vi "VISJS Viewer.vi"(4 "Extra Scripts":string, 5 "FileDependency In":map{path, T1}(c390), 6 "Options":string, 7 "OpenWebBrowser(False)":bool, 8 "error in":errorcluster, 9 "Embedd VISJS Librarya in HTMl File(False)":bool, 10 "HTMLFilePath":path, 11 "LibraryDependency":map{path, T3}(c390)) -> (0 "error out":errorcluster, 3 "HTMLFileContent":string)   [LabVIEW 2020, in "VISJS Viewer.lvlib"] (continued)
,g)||A.deactivate()},document.body.addEventListener(\"click\",this._onClick),this._cleanupQueue.push((function(){document.body.removeEventListener(\"click\",A._onClick)}))),this._escListener=function(g){(\"key\"in g?\"Escape\"===g.key:27===g.keyCode)&&A.deactivate()}}He(jf.prototype),jf.current=null,jf.prototype.destroy=function(){var g,t;this.deactivate();var A,e=Rf(cl(g=Zl(t=this._cleanupQueue).call(t,0)).call(g));try{for(e.s();!(A=e.n()).done;){(0,A.value)()}}catch(g){e.e(g)}finally{e.f()}},jf.prototype.activate=function(){jf.current&&jf.current.deactivate(),jf.current=this,this.active=!0,this._dom.overlay.style.display=\"none\",this._dom.container.classList.add(\"vis-active\"),this.emit(\"change\"),this.emit(\"activate\"),document.body.addEventListener(\"keydown\",this._escListener)},jf.prototype.deactivate=function(){this.active=!1,this._dom.overlay.style.display=\"block\",this._dom.container.classList.remove(\"vis-active\"),document.body.removeEventListener(\"keydown\",this._escListener),this.emit(\"change\"),this.emit(\"deactivate\")},jf.prototype._onTapOverlay=function(g){this.activate(),g.srcEvent.stopPropagation()};var Lf=/^#?([a-f\\d]{2})([a-f\\d]{2})([a-f\\d]{2})$/i,Vf=/^#?([a-f\\d])([a-f\\d])([a-f\\d])$/i,Yf=/^rgb\\( *(1?\\d{1,2}|2[0-4]\\d|25[0-5]) *, *(1?\\d{1,2}|2[0-4]\\d|25[0-5]) *, *(1?\\d{1,2}|2[0-4]\\d|25[0-5]) *\\)$/i,Wf=/^rgba\\( *(1?\\d{1,2}|2[0-4]\\d|25[0-5]) *, *(1?\\d{1,2}|2[0-4]\\d|25[0-5]) *, *(1?\\d{1,2}|2[0-4]\\d|25[0-5]) *, *([01]|0?\\.\\d+) *\\)$/i;function Qf(g){if(g)for(;!0===g.hasChildNodes();){var t=g.firstChild;t&&(Qf(t),g.removeChild(t))}}function Uf(g){return g instanceof String||\"string\"==typeof g}function _f(g){return\"object\"===yd(g)&&null!==g}function Kf(g,t,A,e){var C=!1;!0===e&&(C=null===t[A]&&void 0!==g[A]),C?delete g[A]:g[A]=t[A]}function Hf(g,t){var A=arguments.length>2&&void 0!==arguments[2]&&arguments[2];for(var e in g)if(void 0!==t[e])if(null===t[e]||\"object\"!==yd(t[e]))Kf(g,t,e,A);else{var C=g[e],I=t[e];_f(C)&&_f(I)&&Hf(C,I,A)}}function Xf(g,t,A){var e=arguments.length>3&&void 0!==arguments[3]&&arguments[3];if(Rh(A))throw new TypeError(\"Arrays are not supported by deepExtend\");for(var C=0;C<g.length;C++){var I=g[C];if(Object.prototype.hasOwnProperty.call(A,I))if(A[I]&&A[I].constructor===Object)void 0===t[I]&&(t[I]={}),t[I].constructor===Object?qf(t[I],A[I],!1,e):Kf(t,A,I,e);else{if(Rh(A[I]))throw new TypeError(\"Arrays are not supported by deepExtend\");Kf(t,A,I,e)}}return t}function Jf(g,t,A){var e=arguments.length>3&&void 0!==arguments[3]&&arguments[3];if(Rh(A))throw new TypeError(\"Arrays are not supported by deepExtend\");for(var C in A)if(Object.prototype.hasOwnProperty.call(A,C)&&!Ic(g).call(g,C))if(A[C]&&A[C].constructor===Object)void 0===t[C]&&(t[C]={}),t[C].constructor===Object?qf(t[C],A[C]):Kf(t,A,C,e);else if(Rh(A[C])){t[C]=[];for(var I=0;I<A[C].length;I++)t[C].push(A[C][I])}else Kf(t,A,C,e);return t}function qf(g,t){var A=arguments.length>2&&void 0!==arguments[2]&&arguments[2],e=arguments.length>3&&void 0!==arguments[3]&&arguments[3];for(var C in t)if(Object.prototype.hasOwnProperty.call(t,C)||!0===A)if(\"object\"===yd(t[C])&&null!==t[C]&&sc(t[C])===Object.prototype)void 0===g[C]?g[C]=qf({},t[C],A):\"object\"===yd(g[C])&&null!==g[C]&&sc(g[C])===Object.prototype?qf(g[C],t[C],A):Kf(g,t,C,e);else if(Rh(t[C])){var I;g[C]=wh(I=t[C]).call(I)}else Kf(g,t,C,e);return g}function $f(g,t){var A;return bh(A=[]).call(A,ch(g),[t])}function gv(g){return g.getBoundingClientRect().top}function tv(g,t){if(Rh(g))for(var A=g.length,e=0;e<A;e++)t(g[e],e,g);else for(var C in g)Object.prototype.hasOwnProperty.call(g,C)&&t(g[C],C,g)}function Av(g){var t;switch(g.length){case 3:case 4:return(t=Vf.exec(g))?{r:Gc(t[1]+t[1],16),g:Gc(t[2]+t[2],16),b:Gc(t[3]+t[3],16)}:null;case 6:case 7:return(t=Lf.exec(g))?{r:Gc(t[1],16),g:Gc(t[2],16),b:Gc(t[3],16)}:null;default:return null}}function ev(g,t){if(Ic(g).call(g,\"rgba\"))return g;if(Ic(g).call(g,\"rgb\")){var A=g.substr(Xc(g).call(g,\"(\")+1).replace(\")\",\"\").split(\",\");return\"rgba(\"+A[0]+\",\"+A[1]+\",\"+A[2]+\",\"+t+\")\"}var e=Av(g);return null==e?g:\"rgba(\"+e.r+\",\"+e.g+\",\"+e.b+\",\"+t+\")\"}function Cv(g,t,A){var e;return\"#\"+wh(e=((1<<24)+(g<<16)+(t<<8)+A).toString(16)).call(e,1)}function Iv(g,t){if(Uf(g)){var A=g;if(sv(A)){var e,C=Fh(e=A.substr(4).substr(0,A.length-5).split(\",\")).call(e,(function(g){return Gc(g)}));A=Cv(C[0],C[1],C[2])}if(!0===rv(A)){var I=function(g){var t=Av(g);if(!t)throw new TypeError(\"'\".concat(g,\"' is not a valid color.\"));return iv(t.r,t.g,t.b)}(A),i={h:I.h,s:.8*I.s,v:Math.min(1,1.02*I.v)},o={h:I.h,s:Math.min(1,1.25*I.s),v:.8*I.v},n=nv(o.h,o.s,o.v),r=nv(i.h,i.s,i.v);return{background:A,border:n,highlight:{background:r,border:n},hover:{background:r,border:n}}}return{background:A,border:A,highlight:{background:A,border:A},hover:{background:A,border:A}}}return t?{background:g.background||t.background,border:g.border||t.border,highlight:Uf(g.highlight)?{border:g.highlight,background:g.highlight}:{background:g.highlight&&g.highlight.background||t.highlight.background,border:g.highlight&&g.highlight.border||t.highlight.border},hover:Uf(g.hover)?{border:g.hover,background:g.hover}:{border:g.hover&&g.hover.border||t.hover.border,background:g.hover&&g.hover.background||t.hover.background}}:{background:g.background||void 0,border:g.border||void 0,highlight:Uf(g.highlight)?{border:g.highlight,background:g.highlight}:{background:g.highlight&&g.highlight.background||void 0,border:g.highlight&&g.highlight.border||void 0},hover:Uf(g.hover)?{border:g.hover,background:g.hover}:{border:g.hover&&g.hover.border||void 0,background:g.hover&&g.hover.background||void 0}}}function iv(g,t,A){g/=255,t/=255,A/=255;var e=Math.min(g,Math.min(t,A)),C=Math.max(g,Math.max(t,A));return e===C?{h:0,s:0,v:e}:{h:60*((g===e?3:A===e?1:5)-(g===e?t-A:A===e?g-t:A-g)/(C-e))/360,s:(C-e)/C,v:C}}function ov(g,t,A){var e,C,I,i=Math.floor(6*g),o=6*g-i,n=A*(1-t),r=A*(1-o*t),s=A*(1-(1-o)*t);switch(i%6){case 0:e=A,C=s,I=n;break;case 1:e=r,C=A,I=n;break;case 2:e=n,C=A,I=s;break;case 3:e=n,C=r,I=A;break;case 4:e=s,C=n,I=A;break;case 5:e=A,C=n,I=r}return{r:Math.floor(255*e),g:Math.floor(255*C),b:Math.floor(255*I)}}function nv(g,t,A){var e=ov(g,t,A);return Cv(e.r,e.g,e.b)}function rv(g){return/(^#[0-9A-F]{6}$)|(^#[0-9A-F]{3}$)/i.test(g)}function sv(g){return Yf.test(g)}function av(g){if(null===g||\"object\"!==yd(g))return null;if(g instanceof Element)return g;var t=$c(g);for(var A in g)Object.prototype.hasOwnProperty.call(g,A)&&\"object\"==yd(g[A])&&(t[A]=av(g[A]));return t}function dv(g,t,A){var e=arguments.length>3&&void 0!==arguments[3]?arguments[3]:{},C=function(g){return null!=g},I=function(g){return null!==g&&\"object\"===yd(g)};if(!I(g))throw new Error(\"Parameter mergeTarget must be an object\");if(!I(t))throw new Error(\"Parameter options must be an object\");if(!C(A))throw new Error(\"Parameter option must have a value\");if(!I(e))throw new Error(\"Parameter globalOptions must be an object\");var i=t[A],o=I(e)&&!function(g){for(var t in g)if(Object.prototype.hasOwnProperty.call(g,t))return!1;return!0}(e)?e[A]:void 0,n=o?o.enabled:void 0;if(void 0!==i){if(\"boolean\"==typeof i)return I(g[A])||(g[A]={}),void(g[A].enabled=i);if(null===i&&!I(g[A])){if(!C(o))return;g[A]=$c(o)}if(I(i)){var r=!0;void 0!==i.enabled?r=i.enabled:void 0!==n&&(r=o.enabled),function(g,t,A){I(g[A])||(g[A]={});var e=t[A],C=g[A];for(var i in e)Object.prototype.hasOwnProperty.call(e,i)&&(C[i]=e[i])}(g,t,A),g[A].enabled=r}}}var hv={linear:function(g){return g},easeInQuad:function(g){return g*g},easeOutQuad:function(g){return g*(2-g)},easeInOutQuad:function(g){return g<.5?2*g*g:(4-2*g)*g-1},easeInCubic:function(g){return g*g*g},easeOutCubic:function(g){return--g*g*g+1},easeInOutCubic:function(g){return g<.5?4*g*g*g:(g-1)*(2*g-2)*(2*g-2)+1},easeInQuart:function(g){return g*g*g*g},easeOutQuart:function(g){return 1- --g*g*g*g},easeInOutQuart:function(g){return g<.5?8*g*g*g*g:1-8*--g*g*g*g},easeInQuint:function(g){return g*g*g*g*g},easeOutQuint:function(g){return 1+--g*g*g*g*g},easeInOutQuint:function(g){return g<.5?16*g*g*g*g*g:1+16*--g*g*g*g*g}};function lv(g,t){var A;Rh(t)||(t=[t]);var e,C=Rf(g);try{for(C.s();!(e=C.n()).done;){var I=e.value;if(I){A=I[t[0]];for(var i=1;i<t.length;i++)A&&(A=A[t[i]]);if(void 0!==A)break}}}catch(g){C.e(g)}finally{C.f()}return A}var cv={black:\"#000000\",navy:\"#000080\",darkblue:\"#00008B\",mediumblue:\"#0000CD\",blue:\"#0000FF\",darkgreen:\"#006400\",green:\"#008000\",teal:\"#008080\",darkcyan:\"#008B8B\",deepskyblue:\"#00BFFF\",darkturquoise:\"#00CED1\",mediumspringgreen:\"#00FA9A\",lime:\"#00FF00\",springgreen:\"#00FF7F\",aqua:\"#00FFFF\",cyan:\"#00FFFF\",midnightblue:\"#191970\",dodgerblue:\"#1E90FF\",lightseagreen:\"#20B2AA\",forestgreen:\"#228B22\",seagreen:\"#2E8B57\",darkslategray:\"#2F4F4F\",limegreen:\"#32CD32\",mediumseagreen:\"#3CB371\",turquoise:\"#40E0D0\",royalblue:\"#4169E1\",steelblue:\"#4682B4\",darkslateblue:\"#483D8B\",mediumturquoise:\"#48D1CC\",indigo:\"#4B0082\",darkolivegreen:\"#556B2F\",cadetblue:\"#5F9EA0\",cornflowerblue:\"#6495ED\",mediumaquamarine:\"#66CDAA\",dimgray:\"#696969\",slateblue:\"#6A5ACD\",olivedrab:\"#6B8E23\",slategray:\"#708090\",lightslategray:\"#778899\",mediumslateblue:\"#7B68EE\",lawngreen:\"#7CFC00\",chartreuse:\"#7FFF00\",aquamarine:\"#7FFFD4\",maroon:\"#800000\",purple:\"#800080\",olive:\"#808000\",gray:\"#808080\",skyblue:\"#87CEEB\",lightskyblue:\"#87CEFA\",blueviolet:\"#8A2BE2\",darkred:\"#8B0000\",darkmagenta:\"#8B008B\",saddlebrown:\"#8B4513\",darkseagreen:\"#8FBC8F\",lightgreen:\"#90EE90\",mediumpurple:\"#9370D8\",darkviolet:\"#9400D3\",palegreen:\"#98FB98\",darkorchid:\"#9932CC\",yellowgreen:\"#9ACD32\",sienna:\"#A0522D\",brown:\"#A52A2A\",darkgray:\"#A9A9A9\",lightblue:\"#ADD8E6\",greenyellow:\"#ADFF2F\",paleturquoise:\"#AFEEEE\",lightsteelblue:\"#B0C4DE\",powderblue:\"#B0E0E6\",firebrick:\"#B22222\",darkgoldenrod:\"#B8860B\",mediumorchid:\"#BA55D3\",rosybrown:\"#BC8F8F\",darkkhaki:\"#BDB76B\",silver:\"#C0C0C0\",mediumvioletred:\"#C71585\",indianred:\"#CD5C5C\",peru:\"#CD853F\",chocolate:\"#D2691E\",tan:\"#D2B48C\",lightgrey:\"#D3D3D3\",palevioletred:\"#D87093\",thistle:\"#D8BFD8\",orchid:\"#DA70D6\",goldenrod:\"#DAA520\",crimson:\"#DC143C\",gainsboro:\"#DCDCDC\",plum:\"#DDA0DD\",burlywood:\"#DEB887\",lightcyan:\"#E0FFFF\",lavender:\"#E6E6FA\",darksalmon:\"#E9967A\",violet:\"#EE82EE\",palegoldenrod:\"#EEE8AA\",lightcoral:\"#F08080\",khaki:\"#F0E68C\",aliceblue:\"#F0F8FF\",honeydew:\"#F0FFF0\",azure:\"#F0FFFF\",sandybrown:\"#F4A460\",wheat:\"#F5DEB3\",beige:\"#F5F5DC\",whitesmoke:\"#F5F5F5\",mintcream:\"#F5FFFA\",ghostwhite:\"#F8F8FF\",salmon:\"#FA8072\",antiquewhite:\"#FAEBD7\",linen:\"#FAF0E6\",lightgoldenrodyellow:\"#FAFAD2\",oldlace:\"#FDF5E6\",red:\"#FF0000\",fuchsia:\"#FF00FF\",magenta:\"#FF00FF\",deeppink:\"#FF1493\",orangered:\"#FF4500\",tomato:\"#FF6347\",hotpink:\"#FF69B4\",coral:\"#FF7F50\",darkorange:\"#FF8C00\",lightsalmon:\"#FFA07A\",orange:\"#FFA500\",lightpink:\"#FFB6C1\",pink:\"#FFC0CB\",gold:\"#FFD700\",peachpuff:\"#FFDAB9\",navajowhite:\"#FFDEAD\",moccasin:\"#FFE4B5\",bisque:\"#FFE4C4\",mistyrose:\"#FFE4E1\",blanchedalmond:\"#FFEBCD\",papayawhip:\"#FFEFD5\",lavenderblush:\"#FFF0F5\",seashell:\"#FFF5EE\",cornsilk:\"#FFF8DC\",lemonchiffon:\"#FFFACD\",floralwhite:\"#FFFAF0\",snow:\"#FFFAFA\",yellow:\"#FFFF00\",lightyellow:\"#FFFFE0\",ivory:\"#FFFFF0\",white:\"#FFFFFF\"},uv=function(){function g(){var t=arguments.length>0&&void 0!==arguments[0]?arguments[0]:1;cn(this,g),this.pixelRatio=t,this.generated=!1,this.centerCoordinates={x:144.5,y:144.5},this.r=289*.49,this.color={r:255,g:255,b:255,a:1},this.hueCircle=void 0,this.initialColor={r:255,g:255,b:255,a:1},this.previousColor=void 0,this.applied=!1,this.updateCallback=function(){},this.closeCallback=function(){},this._create()}return kd(g,[{key:\"insertTo\",value:function(g){void 0!==this.hammer&&(this.hammer.destroy(),this.hammer=void 0),this.container=g,this.container.appendChild(this.frame),this._bindHammer(),this._setSize()}},{key:\"setUpdateCallback\",value:function(g){if(\"function\"!=typeof g)throw new Error(\"Function attempted to set as colorPicker update callback is not a function.\");this.updateCallback=g}},{key:\"setCloseCallback\",value:function(g){if(\"function\"!=typeof g)throw new Error(\"Function attempted to set as colorPicker closing callback is not a function.\");this.closeCallback=g}},{key:\"_isColorString\",value:function(g){if(\"string\"==typeof g)return cv[g]}},{key:\"setColor\",value:function(g){var t=!(arguments.length>1&&void 0!==arguments[1])||arguments[1];if(\"none\"!==g){var A,e=this._isColorString(g);if(void 0!==e&&(g=e),!0===Uf(g)){if(!0===sv(g)){var C=g.substr(4).substr(0,g.length-5).split(\",\");A={r:C[0],g:C[1],b:C[2],a:1}}else if(!0===function(g){return Wf.test(g)}(g)){var I=g.substr(5).substr(0,g.length-6).split(\",\");A={r:I[0],g:I[1],b:I[2],a:I[3]}}else if(!0===rv(g)){var i=Av(g);A={r:i.r,g:i.g,b:i.b,a:1}}}else if(g instanceof Object&&void 0!==g.r&&void 0!==g.g&&void 0!==g.b){var o=void 0!==g.a?g.a:\"1.0\";A={r:g.r,g:g.g,b:g.b,a:o}}if(void 0===A)throw new Error(\"Unknown color passed to the colorPicker. Supported are strings: rgb, hex, rgba. Object: rgb ({r:r,g:g,b:b,[a:a]}). Supplied: \"+eu(g));this._setColor(A,t)}}},{key:\"show\",value:function(){void 0!==this.closeCallback&&(this.closeCallback(),this.closeCallback=void 0),this.applied=!1,this.frame.style.display=\"block\",this._generateHueCircle()}},{key:\"_hide\",value:function(){var g=this;!0===(!(arguments.length>0&&void 0!==arguments[0])||arguments[0])&&(this.previousColor=fe({},this.color)),!0===this.applied&&this.updateCallback(this.initialColor),this.frame.style.display=\"none\",wu((function(){void 0!==g.closeCallback&&(g.closeCallback(),g.closeCallback=void 0)}),0)}},{key:\"_save\",value:function(){this.updateCallback(this.color),this.applied=!1,this._hide()}},{key:\"_apply\",value:function(){this.applied=!0,this.updateCallback(this.color),this._updatePicker(this.color)}},{key:\"_loadLast\",value:function(){void 0!==this.previousColor?this.setColor(this.previousColor,!1):alert(\"There is no last color to load...\")}},{key:\"_setColor\",value:function(g){!0===(!(arguments.length>1&&void 0!==arguments[1])||arguments[1])&&(this.initialColor=fe({},g)),this.color=g;var t=iv(g.r,g.g,g.b),A=2*Math.PI,e=this.r*t.s,C=this.centerCoordinates.x+e*Math.sin(A*t.h),I=this.centerCoordinates.y+e*Math.cos(A*t.h);this.colorPickerSelector.style.left=C-.5*this.colorPickerSelector.clientWidth+\"px\",this.colorPickerSelector.style.top=I-.5*this.colorPickerSelector.clientHeight+\"px\",this._updatePicker(g)}},{key:\"_setOpacity\",value:function(g){this.color.a=g/100,this._updatePicker(this.color)}},{key:\"_setBrightness\",value:function(g){var t=iv(this.color.r,this.color.g,this.color.b);t.v=g/100;var A=ov(t.h,t.s,t.v);A.a=this.color.a,this.color=A,this._updatePicker()}},{key:\"_updatePicker\",value:function(){var g=arguments.length>0&&void 0!==arguments[0]?arguments[0]:this.color,t=iv(g.r,g.g,g.b),A=this.colorPickerCanvas.getContext(\"2d\");void 0===this.pixelRation&&(this.pixelRatio=(window.devicePixelRatio||1)/(A.webkitBackingStorePixelRatio||A.mozBackingStorePixelRatio||A.msBackingStorePixelRatio||A.oBackingStorePixelRatio||A.backingStorePixelRatio||1)),A.setTransform(this.pixelRatio,0,0,this.pixelRatio,0,0);var e=this.colorPickerCanvas.clientWidth,C=this.colorPickerCanvas.clientHeight;A.clearRect(0,0,e,C),A.putImageData(this.hueCircle,0,0),A.fillStyle=\"rgba(0,0,0,\"+(1-t.v)+\")\",A.circle(this.centerCoordinates.x,this.centerCoordinates.y,this.r),Bu(A).call(A),this.brightnessRange.value=100*t.v,this.opacityRange.value=100*g.a,this.initialColorDiv.style.backgroundColor=\"rgba(\"+this.initialColor.r+\",\"+this.initialColor.g+\",\"+this.initialColor.b+\",\"+this.initialColor.a+\")\",this.newColorDiv.style.backgroundColor=\"rgba(\"+this.color.r+\",\"+this.color.g+\",\"+this.color.b+\",\"+this.color.a+\")\"}},{key:\"_setSize\",value:function(){this.colorPickerCanvas.style.width=\"100%\",this.colorPickerCanvas.style.height=\"100%\",this.colorPickerCanvas.width=289*this.pixelRatio,this.colorPickerCanvas.height=289*this.pixelRatio}},{key:\"_create\",value:function(){var g,t,A,e;if(this.frame=document.createElement(\"div\"),this.frame.className=\"vis-color-picker\",this.colorPickerDiv=document.createElement(\"div\"),this.colorPickerSelector=document.createElement(\"div\"),this.colorPickerSelector.className=\"vis-selector\",this.colorPickerDiv.appendChild(this.colorPickerSelector),this.colorPickerCanvas=document.createElement(\"canvas\"),this.colorPickerDiv.appendChild(this.colorPickerCanvas),this.colorPickerCanvas.getContext){var C=this.colorPickerCanvas.getContext(\"2d\");this.pixelRatio=(window.devicePixelRatio||1)/(C.webkitBackingStorePixelRatio||C.mozBackingStorePixelRatio||C.msBackingStorePixelRatio||C.oBackingStorePixelRatio||C.backingStorePixelRatio||1),this.colorPickerCanvas.getContext(\"2d\").setTransform(this.pixelRatio,0,0,this.pixelRatio,0,0)}else{var I=document.createElement(\"DIV\");I.style.color=\"red\",I.style.fontWeight=\"bold\",I.style.padding=\"10px\",I.innerText=\"Error: your browser does not support HTML canvas\",this.colorPickerCanvas.appendChild(I)}this.colorPickerDiv.className=\"vis-color\",this.opacityDiv=document.createElement(\"div\"),this.opacityDiv.className=\"vis-opacity\",this.brightnessDiv=document.createElement(\"div\"),this.brightnessDiv.className=\"vis-brightness\",this.arrowDiv=document.createElement(\"div\"),this.arrowDiv.className=\"vis-arrow\",this.opacityRange=document.createElement(\"input\");try{this.opacityRange.type=\"range\",this.opacityRange.min=\"0\",this.opacityRange.max=\"100\"}catch(g){}this.opacityRange.value=\"100\",this.opacityRange.className=\"vis-range\",this.brightnessRange=document.createElement(\"input\");try{this.brightnessRange.type=\"range\",this.brightnessRange.min=\"0\",this.brightnessRange.max=\"100\"}catch(g){}this.brightnessRange.value=\"100\",this.brightnessRange.className=\"vis-range\",this.opacityDiv.appendChild(this.opacityRange),this.brightnessDiv.appendChild(this.brightnessRange);var i=this;this.opacityRange.onchange=function(){i._setOpacity(this.value)},this.opacityRange.oninput=function(){i._setOpacity(this.value)},this.brightnessRange.onchange=function(){i._setBrightness(this.value)},this.brightnessRange.oninput=function(){i._setBrightness(this.value)},this.brightnessLabel=document.createElement(\"div\"),this.brightnessLabel.className=\"vis-label vis-brightness\",this.brightnessLabel.innerText=\"brightness:\",this.opacityLabel=document.createElement(\"div\"),this.opacityLabel.className=\"vis-label vis-opacity\",this.opacityLabel.innerText=\"opacity:\",this.newColorDiv=document.createElement(\"div\"),this.newColorDiv.className=\"vis-new-color\",this.newColorDiv.innerText=\"new\",this.initialColorDiv=document.createElement(\"div\"),this.initialColorDiv.className=\"vis-initial-color\",this.initialColorDiv.innerText=\"initial\",this.cancelButton=document.createElement(\"div\"),this.cancelButton.className=\"vis-button vis-cancel\",this.cancelButton.innerText=\"cancel\",this.cancelButton.onclick=je(g=this._hide).call(g,this,!1),this.applyButton=document.createElement(\"div\"),this.applyButton.className=\"vis-button vis-apply\",this.applyButton.innerText=\"apply\",this.applyButton.onclick=je(t=this._apply).call(t,this),this.saveButton=document.createElement(\"div\"),this.saveButton.className=\"vis-button vis-save\",this.saveButton.innerText=\"save\",this.saveButton.onclick=je(A=this._save).call(A,this),this.loadButton=document.createElement(\"div\"),this.loadButton.className=\"vis-button vis-load\",this.loadButton.innerText=\"load last\",this.loadButton.onclick=je(e=this._loadLast).call(e,this),this.frame.appendChild(this.colorPickerDiv),this.frame.appendChild(this.arrowDiv),this.frame.appendChild(this.brightnessLabel),this.frame.appendChild(this.brightnessDiv),this.frame.appendChild(this.opacityLabel),
